vi "Toggle Menu Items.vi"(7 "Item Tag":string, 8 "error in (no error)":errorcluster, 9 "Item Index":i32, 10 "Menu Ref":refnum<k9>, 11 "KIT-QA in":refnum<class "KIT-QA.lvclass">) -> (0 "error out":errorcluster, 3 "KIT-QA out":refnum<class "KIT-QA.lvclass">)   [LabVIEW 2016, in "KIT-QA.lvlib" / "KIT-QA.lvclass"]
doc: "Toggle set of selected channels."
uses:
  KIT-QA.lvclass
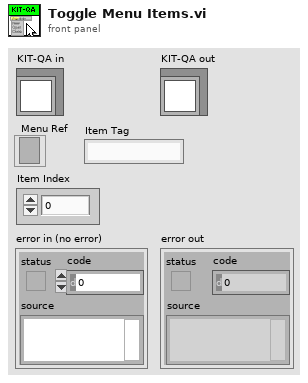
[diagram p1: front panel]
types:
  T1 = typedef "LVMenuShortCut.ctl" = cluster{"include Shift key?":bool, "include Ctrl key?":bool, "shortcut key":string}
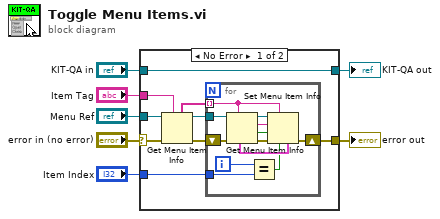
[diagram p0: block diagram]
diagram:
  n1 = case shown="No Error" "error in (no error)" {
    selector: "error in (no error)" -> [w12 w30]
    tunnel: [w15 w30] -> w6
    tunnel: [w16 w29] -> w4
    tunnel: "KIT-QA in" -> [w16 w29]
    tunnel: "Menu Ref" -> [w13 _]
    tunnel: "Item Index" -> [w14 _]
    tunnel: "Item Tag" -> [w8 _]
    frame No Error {
      n2 = Get Menu Item Info(7:w8, 8:w12, 11:w13) -> (0:w9:errorcluster, 3:w10:refnum<k9>, 5:w11:string[])  [unwired: 4 out]
      n3 = for {
        tunnel: w11 -> [w24] mode=indexing
        tunnel: w10 -> [w27]
        shift-right: [w18] -> w15
        shift-left: w9 -> [w28]
        tunnel: w14 -> [w17]
        i -> [w20]
        n4 = Get Menu Item Info(7:w24, 8:w28, 11:w27) -> (0:w25:errorcluster, 1:w22:bool, 2:w23:string, 3:w26:refnum<k9>, 6:w21:T1)  [unwired: 2 out]
        n5 = Equal?(x=w20, y=w17) -> (x = y?=w19:bool)
        n6 = Set Menu Item Info(4:w21, 6:w19, 7:w24, 8:w25, 9:w22, 10:w23, 11:w26) -> (0:w18:errorcluster)  [unwired: 1 out]
      }
    }
    frame Error {
    }
  }
  "error out" <- w6
  "KIT-QA out" <- w4
